vi "LinearVelocity.vi"(10 "Velocity":dbl, 11 "LineArray":cluster{"X":dbl, "Y":dbl, "OnOff":bool}[](array[cluster])) -> (0 "XY Graph":cluster{"X":dbl, "Y":dbl}[](graph), 2 "Yvelocities":T1(array[cluster]), 3 "Xvelocities":T2(array[cluster]))   [LabVIEW 2014]
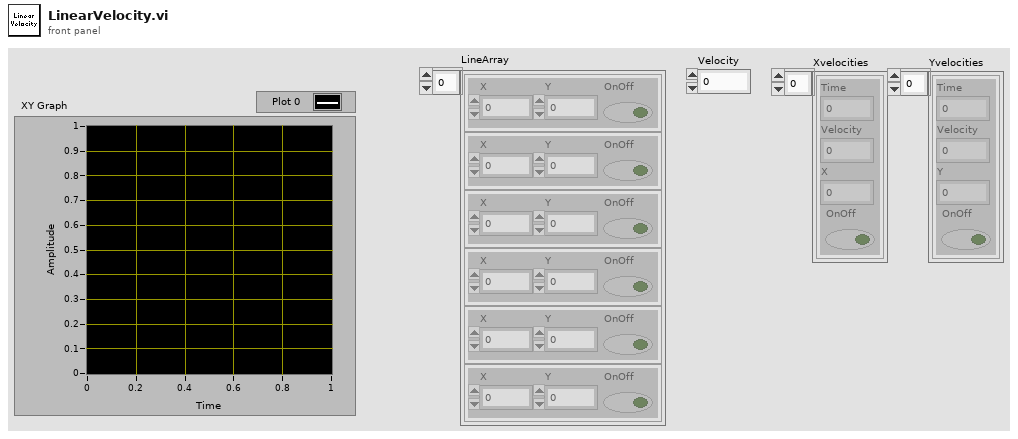
[diagram p1: front panel]
types:
  T1 = cluster{"Time":dbl, "Velocity":dbl, "Y":dbl, "OnOff":bool}[]
  T2 = cluster{"Time":dbl, "Velocity":dbl, "X":dbl, "OnOff":bool}[]
  T3 = cluster{"Time":dbl, "Velocity":dbl, "Position":dbl, "On/Off":bool}
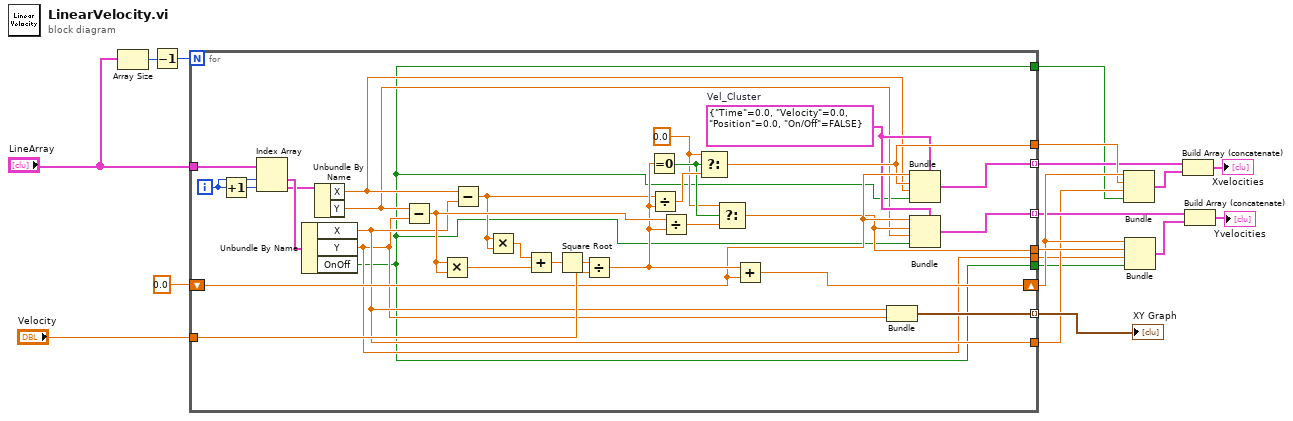
[diagram p0: block diagram]
diagram:
  n1 = Array Size(array="LineArray") -> (size(s)=w19:i32)
  n2 = Decrement(x=w19) -> (x-1=w18:i32)
  n3 = for {
    N: w18 -> [_]
    tunnel: "LineArray" -> [w49]
    tunnel: "Velocity" -> [w44]
    tunnel: [w40] -> w17 mode=indexing
    shift-right: [w33] -> w14
    shift-left: 0.0 -> [w32]
    tunnel: [w31] -> w10 mode=indexing
    tunnel: [w30] -> w12 mode=indexing
    tunnel: [w29] -> w15
    tunnel: [w28] -> w13
    tunnel: [w23] -> w8
    tunnel: [w21] -> w7
    tunnel: [w20] -> w2
    tunnel: [w20] -> w1
    i -> [w46]
    w25 = T3 {"Time"=0.0, "Velocity"=0.0, "Position"=0.0, "On/Off"=FALSE}  # Vel_Cluster
    w35 = 0.0
    n4 = Increment(x=w46) -> (x+1=w47:i32)
    n5 = Index Array(array=w49, index #1=w46, index #2=w47) -> (element #1=w48:cluster{"X":dbl, "Y":dbl, "OnOff":bool}, element #2=w45:cluster{"X":dbl, "Y":dbl, "OnOff":bool})
    n6 = Unbundle By Name(w48) -> ("X"=w23:dbl, "Y"=w21:dbl, "OnOff"=w20:bool)
    n7 = Unbundle By Name(w45) -> ("X"=w24:dbl, "Y"=w22:dbl)
    n8 = Subtract(x=w22, y=w21) -> (x-y=w41:dbl)
    n9 = Multiply(x=w41, y=w41) -> (x*y=w42:dbl)
    n10 = Subtract(x=w24, y=w23) -> (x-y=w34:dbl)
    n11 = Multiply(x=w34, y=w34) -> (x*y=w43:dbl)
    n12 = Add(x=w43, y=w42) -> (x+y=w27:dbl)
    n13 = Square Root(x=w27) -> (sqrt(x)=w26:dbl)
    n14 = Divide(x=w26, y=w44) -> (x/y=w38:dbl)
    n15 = Equal To 0?(x=w38) -> (x = 0?=w36:bool)
    n16 = Divide(x=w34, y=w38) -> (x/y=w39:dbl)
    n17 = Divide(x=w41, y=w38) -> (x/y=w37:dbl)
    n18 = Select(t=w35, s=w36, f=w39) -> (s? t:f=w28:dbl)
    n19 = Select(t=w35, s=w36, f=w37) -> (s? t:f=w29:dbl)
    n20 = Add(x=w38, y=w32) -> (x+y=w33:dbl)
    n21 = Bundle("X"=w23, "Y"=w21) -> (w40:cluster{"X":dbl, "Y":dbl})  [unwired: 1 in]
    n22 = Bundle(cluster=w25, "Time"=w32, "Velocity"=w28, "Position"=w24, "On/Off"=w20) -> (w30:T3)
    n23 = Bundle(cluster=w25, "Time"=w32, "Velocity"=w29, "Position"=w22, "On/Off"=w20) -> (w31:T3)
  }
  "XY Graph" <- w17
  n24 = Bundle(w14, w13, "X"=w8, "OnOff"=w2) -> (w11:cluster{dbl, dbl, "X":dbl, "OnOff":bool})  [unwired: 1 in]
  n25 = Bundle(w14, w15, "Y"=w7, "OnOff"=w1) -> (w9:cluster{dbl, dbl, "Y":dbl, "OnOff":bool})  [unwired: 1 in]
  n26 = Build Array (concatenate)(w12, w11) -> (→"Xvelocities":T2)
  n27 = Build Array (concatenate)(w10, w9) -> (→"Yvelocities":T1)
